vi "GetConfig.vi"(8 "error in (no error)":errorcluster, 11 "reference in":refnum<class "niMmWave_Transceiver.lvclass">) -> (0 "error out":errorcluster, 2 "String":string, 3 "reference out":refnum<class "niMmWave_Transceiver.lvclass">)   [LabVIEW 2019, in "niMmWave_Transceiver.lvclass"]
doc: "Returns actual system configuration as JSON string"
uses:
  niMmWave_Transceiver.lvclass
  C:/Barkhausen mmWave radar/Development/modules/mmw_instrument/src_LabVIEW/Host/SubVIs/mmWave instrument_class/mmWave instrument.lvclass
  Shared/Config state.ctl
  mmWave instrument_class/System info.ctl
  mmWave instrument_class/System state.ctl
  mmWave instrument_class/Instrument state.ctl
  mmWave instrument_class/Instrument mode.ctl
  mmWave instrument_class/Sync mode.ctl
  mmWave instrument_class/RF port info.ctl
  mmWave instrument_class/mmWave instrument.lvclass
  <vilib>/addons/_JKI.lib/Serialization/JSON/JKI JSON Serialization.lvlib
  Shared/Shared.lvlib
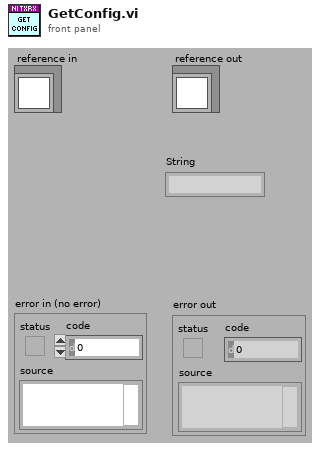
[diagram p1: front panel]
types:
  T1 = typedef "Shared.lvlib/Config state.ctl" = cluster{"system info":T2, "state":T3, "tx":T7, "rx":T7, "versions":cluster{"app":string, "tx fpga":string, "rx fpga":string}}
  T2 = typedef "mmWave instrument.lvclass/System info.ctl" = cluster{"mmw instr":string, "max fs":dbl, "RX/LO1 src":string, "TX/LO1 src":string, "LO2 src":string, "RX LO1 export":bool, "TX LO1 export":bool, "LO2 export":bool, "TX LO1 export level":dbl, "RX LO1 export level":dbl, "LO2 export level":dbl}
  T3 = typedef "mmWave instrument.lvclass/System state.ctl" = cluster{"hw state":T4, "lo sync en":bool, "trig sync en":bool, "mode":T5, "sync":T6, "equalization en":bool}
  T4 = typedef "mmWave instrument.lvclass/Instrument state.ctl" = enum16{"Off", "Initialization", "Configuration", "Running", "Calibration"}
  T5 = typedef "mmWave instrument.lvclass/Instrument mode.ctl" = enum16{"RF", "IF", "BB"}
  T6 = typedef "mmWave instrument.lvclass/Sync mode.ctl" = enum16{"Slave", "Master"}
  T7 = typedef "mmWave instrument.lvclass/RF port info.ctl" = cluster{"fc":dbl, "gain":dbl, "fs":dbl, "trigger delay":dbl}
  T8 = typedef "niMmWave_Transceiver.lvclass/ObjectAttributes.ctl" = cluster{"session":T9[], "HW.RX resources":T23, "RF config":T24, "RX trigger options":T25, "TX trigger options":T25, "RX samples":i32, "Downloaded Bursts":map{string, T28}, "TX Fs":dbl, "RX Fs":dbl, "burst sequence":string[]}
  T9 = typedef "Session.ctl" = cluster{"3620 session":refnum<queue>, "tx baseband session":T10, "rx baseband session":T18, "tx gain (dB)":dbl, "rx gain (dB)":dbl, "hardware configuration":T19, "gain ranging":T21[], "pxi trigger bus information":T22}
  T10 = typedef "Tx Baseband Session.ctl" = cluster{"3610 session":T11, "7902 reference":T17}
  T11 = typedef "ni3610_and_ni3630_Driver_Lib.lvlib/Main Settings.ctl" = cluster{"VISA resource name":refnum<visa-resource-name>, "Address Space":T12, "window_offset":u32, "register_addresses":T13, "required_MM_fpga_version":cluster{"signature":u32, "hardware":u32, "current revision":u32, "oldest revision":u32}, "CPLD Oldest Compat Version ":cluster{"hardware":u32, "CPLD firmware":u32}, "MM_FPGA_image_location":string, "is_init":bool, "card_type":T14, "DacLmkConfigFileName":string, "AdcLmkConfigFileName":string, "AdcConfigFileName":string, "DacConfigFileName_RevA":string, "DacConfigFileName_RevB":string, "Mulde hardware revision":u8, "bypass DAC PLL\n":bool, "IQ Card Revision":T15, "board capability":T16}
  T12 = typedef "VISA Register Access Address Space.ctl" = u16
  T13 = typedef "ni3610_and_ni3630_Driver_Lib.lvlib/Register Adresses.ctl" = cluster{"MM based Registers":cluster{"Revision":u32, "OldestCompatRev":u32, "signature":u32, "scratch":u32, "LedControl":u32, "BoardHwRev":u32, "BoardControl":u32, "ThermalStatus":u32, "BasebandStatus":u32, "BasebandControl":u32, "BasebandAuxSetup":u32, "BasebandAuxStatus":u32, "LmkSyncOutSetup":u32, " AdcSyncOutSetup":u32, " InjSyncOutSetup":u32, " PxiTrig0OutSetup":u32, " PxiTrig1OutSetup":u32, " PxiTrig2OutSetup":u32, " PxiTrig3OutSetup":u32, " PxiTrig4OutSetup":u32, " PxiTrig5OutSetup":u32, " PxiTrig6OutSetup":u32, " PxiTrig7OutSetup":u32}, "CPLD based Registers":cluster{"SlaveSignature":u32, "SlaveRevision":u32, "SlaveOldestCompatRev":u32, "SlaveScratch":u32, "SlaveSetup":u32, "SlaveStatus":u32, "IDacReg_offset":u32, "LMKRegGrp0_offset":u32, "QDacReg_offset":u32, "BrdTempSensorVal":u32, "TempSensorPowerDown":u32, "GPIOReg_offset":u32, "IAdcReg_offset":u32, "QAdcReg_offset":u32, "LMKRegGrp1_offset":u32, "QadcTempSensorVal":u32, "IadcTempSensorVal":u32, "RevisionReg":u32, "VcxoReg":u32, "CpldStatusReg":u32, "PowerReg":u32, "VBiasEnReg":u32, "ExtRefOeReg":u32, "QdacCtrlReg":u32, "QdacStatusReg":u32, "IdacCtrlReg":u32, "IdacStatusReg":u32, "QdacJtagIn":u32, "QdacJtagOut":u32, "IdacJtagIn":u32, "IdacJtagOut":u32, "IqDcSetupReg":u32, "QadcStatusReg":u32, "IadcStatusReg":u32, "BrdSetupReg":u32, "IqDcRevisionReg":u32, "PllStatusReg":u32, "EndpointScratchReg":u32, "AdcSyncCfgReg":u32, "IqCardOpampReg":u32}, "CPLD Register Offset":u32, "MM  Register Offset":u32, " PxiTrig0OutSetup":u32}
  T14 = typedef "ni3610_and_ni3630_Driver_Lib.lvlib/Base Card Type.ctl" = enum16{"unspecified", "ADC", "DAC"}
  T15 = typedef "ni3610_and_ni3630_Driver_Lib.lvlib/IQ Card Revision.ctl" = enum16{"RevA", "RevB", "RevC", "RevD"}
  T16 = typedef "ni3610_and_ni3630_Driver_Lib.lvlib/Board Capability.ctl" = cluster{"baseband sync":enum16{"no baseband sync", "baseband sync"}}
  T17 = typedef "Blank FPGA Reference.ctl" = refnum<k20>
  T18 = typedef "Rx Baseband Session.ctl" = cluster{"3630 session":T11, "7902 reference":T17}
  T19 = typedef "Hardware Configuration.ctl" = cluster{"direction":T20, "baseband only":bool}
  T20 = typedef "Direction.ctl" = enum16{"Transceiver", "Receiver", "Transmitter"}
  T21 = typedef "Gain Ranging.ctl" = cluster{"gain ranging active scope":string, "gain ranging stream session":refnum<k20>}
  T22 = typedef "PXI Trigger Bus Info.ctl" = cluster{"chassis resource name":refnum<visa-resource-name>, "7902R (TX)":i16, "3610 (TX)":i16, "3620 (IF)":i16, "3630 (RX)":i16, "7902R (RX)":i16}
  T23 = typedef "mmWave HW Control.lvlib/HW TXRX resources cluster.ctl" = cluster{"TX_DAC":refnum<visa-resource-name>, "TX_FPGA":tag, "IF":tag, "RX_ADC":refnum<visa-resource-name>, "RX_FPGA":tag}
  T24 = typedef "mmWave HW Control.lvlib/HW TXRX RF config cluster.ctl" = cluster{"TX.Frequency":dbl, "TX.Gain":dbl, "TX.mmWave adapter":string, "RX.Frequency":dbl, "RX.Gain":dbl, "RX.mmWave adapter":string}
  T25 = typedef "TX trigger config.ctl" = cluster{"delay":dbl, "trig source":T26, "PXI src":i32, "export":T27, "PXI dest":i32}
  T26 = typedef "FPGA Utility.lvlib/FPGA driver trigger source.ctl" = enum16{"Use Tclk", "PXI_Trig", "Aurora RX trig"}
  T27 = typedef "FPGA Utility.lvlib/FPGA driver trigger destination.ctl" = enum16{"None", "Source trig", "Synced trig", "Delayed sync"}
  T28 = typedef "niMmWave_Transceiver.lvclass/BurstInfo.ctl" = cluster{"starting addr":u32, "end addr":u32}
  T29 = typedef "mmWave instrument.lvclass/ObjectAttributes.ctl" = cluster{"mode":T5, "instr state":T4, "Max Fs":dbl, "Equalization coeff":cdb[], "LO sync en":bool, "Trig sync en":bool, "LO sources":T30, "LO Export":T31, "Fc.range":cluster{"min":dbl, "max":dbl}, "Sync mode":T6, "equalization en":bool, "sequence":string[]}
  T30 = typedef "mmWave HW Control.lvlib/LO sources.ctl" = cluster{"RX/LO1 src":string, "TX/LO1 src":string, "LO2 src":string}
  T31 = typedef "mmWave HW Control.lvlib/LO export.ctl" = cluster{"TX LO1 export":bool, "TX LO1 export level":dbl, "RX LO1 export":bool, "RX LO1 export level":dbl, "LO2 export":bool, "LO2 export level":dbl}
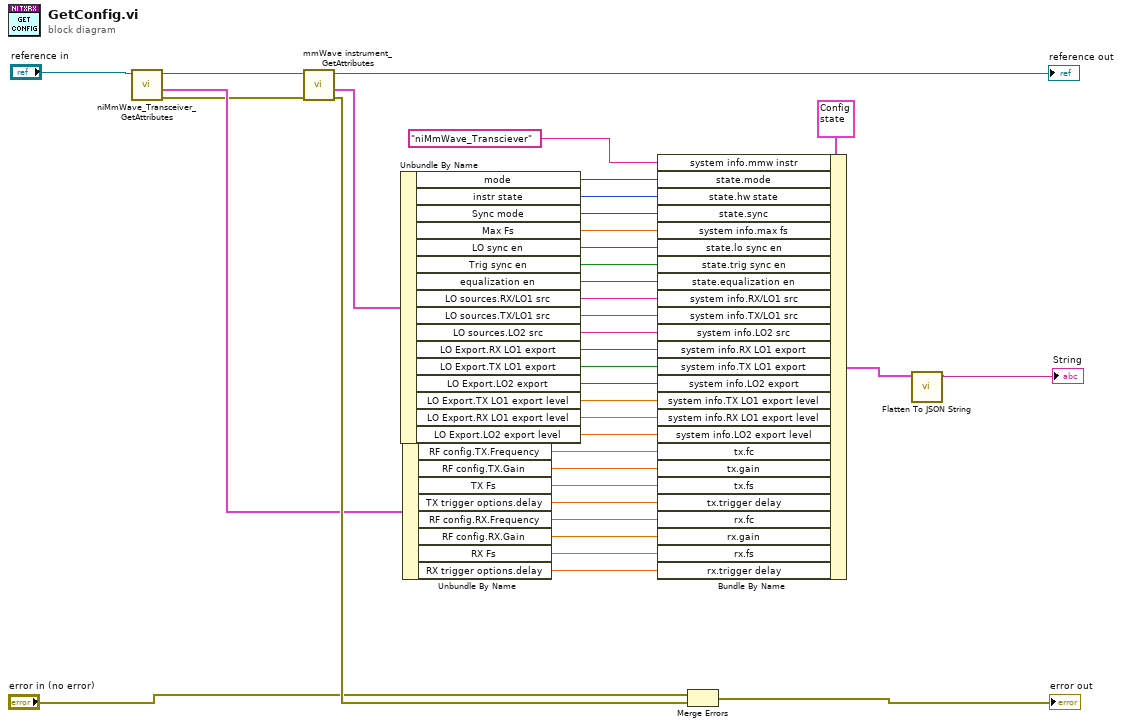
[diagram p0: block diagram]
diagram:
  n1 = call "niMmWave_Transceiver_GetAttributes.vi"("reference in"="reference in") -> ("error out"=w6:errorcluster, "attributes"=w33:T8, "reference out"=w32:refnum<class "niMmWave_Transceiver.lvclass">)  [unwired: 7 in, 1 out]
  n2 = call "mmWave instrument_GetAttributes.vi"("error in (no error)"=w6, "reference in"=w32) -> ("error out"=w37:errorcluster, "attributes"=w31:T29, "reference out"=→"reference out":refnum<class "niMmWave_Transceiver.lvclass">)  [unwired: 6 in, 1 out]
  n3 = Unbundle By Name(w31) -> ("mode"=w29:T5, "instr state"=w28:T4, "Sync mode"=w2:T6, "Max Fs"=w27:dbl, "LO sync en"=w26:bool, "Trig sync en"=w25:bool, "equalization en"=w1:bool, "LO sources.RX/LO1 src"=w24:string, "LO sources.TX/LO1 src"=w23:string, "LO sources.LO2 src"=w22:string, "LO Export.RX LO1 export"=w21:bool, "LO Export.TX LO1 export"=w20:bool, "LO Export.LO2 export"=w19:bool, "LO Export.TX LO1 export level"=w18:dbl, "LO Export.RX LO1 export level"=w17:dbl, "LO Export.LO2 export level"=w16:dbl)
  n4 = Unbundle By Name(w33) -> ("RF config.TX.Frequency"=w15:dbl, "RF config.TX.Gain"=w14:dbl, "TX Fs"=w12:dbl, "TX trigger options.delay"=w13:dbl, "RF config.RX.Frequency"=w11:dbl, "RF config.RX.Gain"=w10:dbl, "RX Fs"=w9:dbl, "RX trigger options.delay"=w8:dbl)
  n5 = Bundle By Name(cluster=T1 {"system info"={"mmw instr"="", "max fs"=0.0, "RX/LO1 src"="", "TX/LO1 src"="", "LO2 src"="", "RX LO1 export"=FALSE, "TX LO1 export"=FALSE, "LO2 export"=FALSE, "TX LO1 export level"=0.0, "RX LO1 export level"=0.0, "LO2 export level"=0.0}, "state"={"hw state"=enum."Off", "lo sync en"=FALSE, "trig sync en"=FALSE, "mode"=enum."RF", "sync"=enum."Slave", "equalization en"=FALSE}, "tx"={"fc"=0.0, "gain"=0.0, "fs"=0.0, "trigger delay"=0.0}, "rx"={"fc"=0.0, "gain"=0.0, "fs"=0.0, "trigger delay"=0.0}, "versions"={"app"="", "tx fpga"="", "rx fpga"=""}} ("Transciever config"), "system info.mmw instr"="niMmWave_Transciever" ("sistem info.mmw instr"), "state.mode"=w29, "state.hw state"=w28, "state.sync"=w2, "system info.max fs"=w27, "state.lo sync en"=w26, "state.trig sync en"=w25, "state.equalization en"=w1, "system info.RX/LO1 src"=w24, "system info.TX/LO1 src"=w23, "system info.LO2 src"=w22, "system info.RX LO1 export"=w21, "system info.TX LO1 export"=w20, "system info.LO2 export"=w19, "system info.TX LO1 export level"=w18, "system info.RX LO1 export level"=w17, "system info.LO2 export level"=w16, "tx.fc"=w15, "tx.gain"=w14, "tx.fs"=w12, "tx.trigger delay"=w13, "rx.fc"=w11, "rx.gain"=w10, "rx.fs"=w9, "rx.trigger delay"=w8) -> (w7:T1)
  n6 = Merge Errors("error in (no error)", w37) -> (→"error out":errorcluster)
  n7 = call <vilib>:"Flatten To JSON String.vi"("Variant"=w7) -> ("JSON String"=→"String":string)  [unwired: 9 in, 1 out]
